vi "cbind.vi"(11 "data":dbl[][](array[numeric])) -> (3 "data (cbind)":dbl[][](array[numeric]))   [LabVIEW 2014]
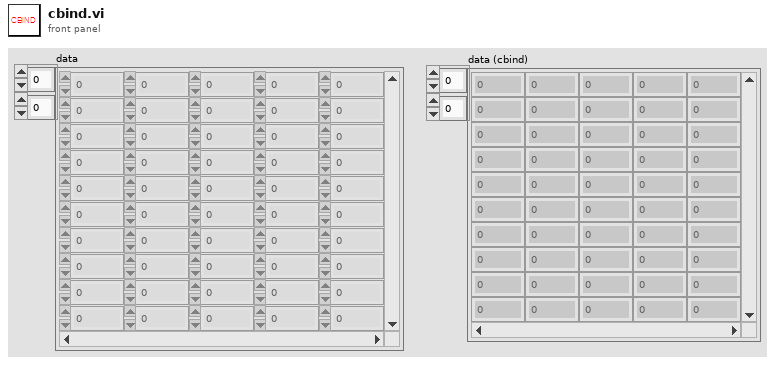
[diagram p1: front panel]
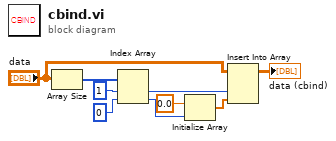
[diagram p0: block diagram]
diagram:
  n1 = Array Size(array="data") -> (size(s)=w2:i32[])
  n2 = Index Array(array=w2, index #1=1 ("index"), index #2=0 ("index")) -> (element #1=w4:i32, element #2=w6:i32)
  n3 = Initialize Array(0.0, w6) -> (w8:dbl[])
  n4 = Insert Into Array(array="data", index (col)=w4, new element=w8) -> (→"data (cbind)":dbl[][])  [unwired: 1 in]
